vi "Get Input Sensor Range.vi"(0 "VISA resource name":refnum<visa-resource-name>, 5 "Channel (1:1)":u16(ring)=1 items=["All (Measurement Inputs)", "1", "2", "3", "4", "5", "6", "7", "8", "9", "10", "11", "12", "13", "14", "15", "16", "A (Control Input)"], 11 "error in (no error)":errorcluster) -> (2 "Preferred Units (1: Kelvin)":u16(ring)=1 items=["Kelvin"=1, "Ohms"=2], 3 "Resistance Range":u16(ring)=21 items=["2.00 mOhm"=1, "6.32 mOhm"=2, "20.0 mOhm"=3, "63.2 mOhm"=4, "200 mOhm"=5, "632 mOhm"=6, "2.00 Ohm"=7, "6.32 Ohm"=8, "20.0 Ohm"=9, "63.2 Ohm"=10, "200 Ohm"=11, "632 Ohm"=12, "2.00 kOhm"=13, "6.32 kOhm"=14, "20.0 kOhm"=15, "63.2 kOhm"=16, "200 kOhm"=17, "632 kOhm"=18, "2.00 MOhm"=19, "6.32 MOhm"=20, "20.0 MOhm"=21, "63.2 MOhm"=22], 4 "VISA resource name out":refnum<visa-resource-name>, 6 "Excitation Mode":u16(ring) items=["Voltage", "Current"], 8 "Excitation Range":u16(ring)=11 items=["2.00 uV / 1.00 pA"=1, "6.32 uV / 3.16 pA"=2, "20.0 uV / 10.0 pA"=3, "63.2 uV / 31.6 pA"=4, "200 uV / 100 pA"=5, "632 uV / 316 pA"=6, "2.00 mV / 1.00 nA"=7, "6.32 mV / 3.16 nA"=8, "20.0 mV / 10.0 nA"=9, "63.2 mV / 31.6 nA"=10, "200 mV / 100 nA"=11, "632 mV / 316 nA"=12, "1.00 uA"=13, "3.16 uA"=14, "10.0 uA"=15, "31.6 uA"=16, "100 uA"=17, "316 uA"=18, "1.00 mA"=19, "3.16 mA"=20, "10.0 mA"=21, "31.6 mA"=22], 10 "Autorange (0: Off)":u16(ring) items=["Autorange off", "Autorange Current", "ROX 102B Autorange"], 14 "Excitation On":bool, 15 "error out":errorcluster)   [LabVIEW 2019, in "Lake Shore 372.lvlib"]
doc: "Queries the Excitation Modes, Resistance Range, and Autorange.\n\nRemarks:\nWhen control input A is selected, the response values get modified to represent the appropriate values in\nthe indicator for Excitation Range.\nResponse Excitation Value \n1 --> 6 \n2 --> 7 \n3 --> 8 \n4 --> 9 \n5 --> 10 \n6 --> 11"
uses:
  Lake Shore 372.lvlib
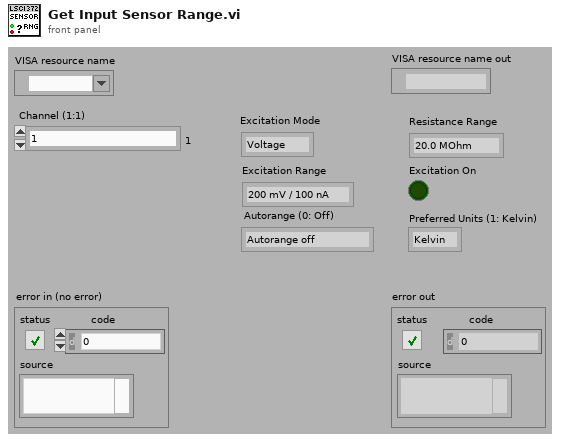
[diagram p1: front panel]
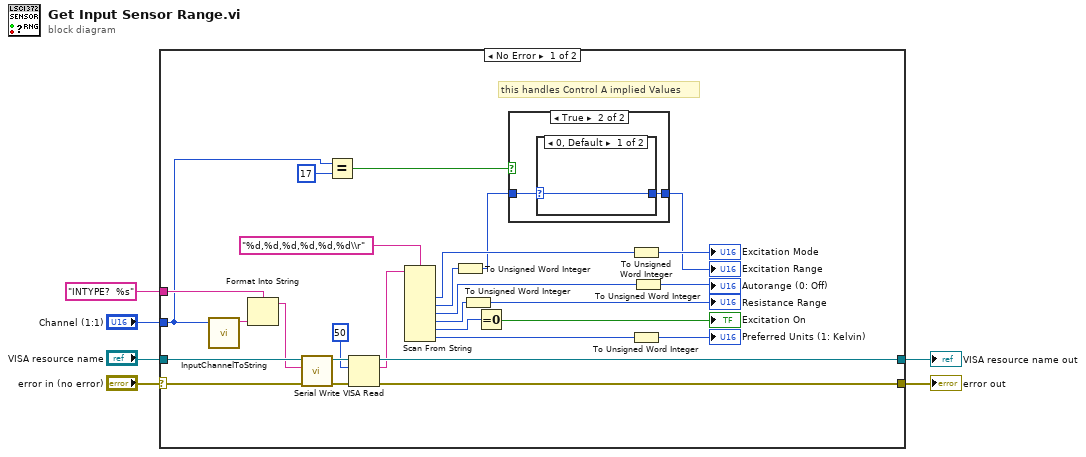
[diagram p0: block diagram]
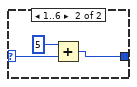
[diagram p3: hidden frame]
diagram:
  n1 = case shown="No Error" "error in (no error)" {
    selector: "error in (no error)" -> [w18 w42]
    tunnel: "VISA resource name" -> [w31 w43]
    tunnel: [w30 w42] -> w5
    tunnel: [w29 w43] -> w4
    tunnel: "INTYPE?  %s" -> [w28 _]
    tunnel: "Channel (1:1)" -> [w16 _]
    frame No Error {
      # "this handles Control A implied Values"
      n2 = call "InputChannelToString.vi"("Channel (1)"=w16) -> ("Channel Str"=w27:string)  [unwired: 10 in]
      n3 = Format Into String(format string=w28, w27) -> (resulting string=w26:string)  [unwired: 2 in, 1 out]
      n4 = call "Serial Write.vi"("error in (no error)"=w18, "Write Buffer (\"\")"=w26, "VISA resource name"=w31) -> ("error out"=w33:errorcluster, "VISA resource name out"=w34:refnum<visa-resource-name>)  [unwired: 6 in, 1 out]
      n5 = Equal?(x=w16, y=u16 17) -> (x = y?=w14:bool)
      n6 = VISA Read(VISA resource name=w34, byte count=50, error in (no error)=w33) -> (VISA resource name out=w29:refnum<visa-resource-name>, read buffer=w24:string, error out=w30:errorcluster)  [unwired: 1 out]
      n7 = Scan From String(format string="%d,%d,%d,%d,%d,%d\\r", input string=w24) -> (output 1=w22:i32, output 2=w21:i32, output 3=w17:i32, output 4=w20:i32, output 5=w23:i32, output 6=w19:i32)  [unwired: 8 in, 3 out]
      n8 = To Unsigned Word Integer(number=w21) -> (unsigned 16bit integer=w13:u16)
      n9 = To Unsigned Word Integer(number=w20) -> (unsigned 16bit integer=→"Resistance Range":u16)
      n10 = Equal To 0?(x=w23) -> (x = 0?=→"Excitation On":bool)
      n11 = case shown="True" w14 {
        tunnel: w13 -> [w35 w37]
        tunnel: [w35 w36] -> w11
        frame False {
        }
        frame True {
          n12 = case shown="0, Default" w37 {
            selector: w37 -> [w38 w41]
            tunnel: [w38 w39] -> w36
            frame 0, Default {
            }
            frame 1..6 {
              n13 = Add(x=u16 5, y=w41) -> (x+y=w39:u16)
            }
          }
        }
      }
      "Excitation Range" <- w11
      n14 = To Unsigned Word Integer(number=w22) -> (unsigned 16bit integer=→"Excitation Mode":u16)
      n15 = To Unsigned Word Integer(number=w19) -> (unsigned 16bit integer=→"Preferred Units (1: Kelvin)":u16)
      n16 = To Unsigned Word Integer(number=w17) -> (unsigned 16bit integer=→"Autorange (0: Off)":u16)
    }
    frame Error {
    }
  }
  "error out" <- w5
  "VISA resource name out" <- w4
